vi "Create and Script 1553 System Definition.vi"(7 "configure logging":bool, 8 "error in":errorcluster, 11 "System Definition Name":string) -> (0 "error out":errorcluster, 2 "log file path":string, 3 "System Definition Path":path)   [LabVIEW 2023]
uses:
  Shared/AIM Hardware Parameters.ctl
  Shared/Initialization Method.ctl
  Shared/Bus Selection.ctl
  Shared/Coupling Mode.ctl
  Shared/Timing Mode.ctl
  <vilib>/NI/VeriStand Custom Device Testing Tools/VeriStandTestUtilities/VeriStandTestUtilities.lvlib
  Scripting/AIM MIL-STD-1553 Scripting.lvlib
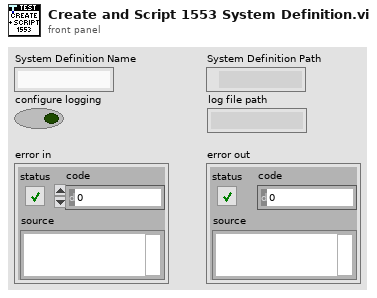
[diagram p1: front panel]
types:
  T1 = typedef "AIM Hardware Parameters.ctl" = cluster{"initialization method":T2, "card number":i32, "pxi slot number":i32, "biu number":i32, "bus selection":T3, "coupling mode":T4, "timing mode":T5}
  T2 = typedef "Initialization Method.ctl" = enum16{"PXI Slot Number", "Card Number"}
  T3 = typedef "Bus Selection.ctl" = enum16{"Both", "Primary", "Secondary"}
  T4 = typedef "Coupling Mode.ctl" = enum16{"Isolated Onboard Termination", "Transformer Coupled", "Direct Coupled", "External with Onboard Termination", "Onboard Digital Wrap-around"}
  T5 = typedef "Timing Mode.ctl" = enum16{"Disabled (Relative Timestamps)", "IRIG (Internal System Time)", "IRIG (External Timing Source)"}
  T6 = typedef "Custom Device API.lvlib/Custom Device Item Ref.ctl" = u64
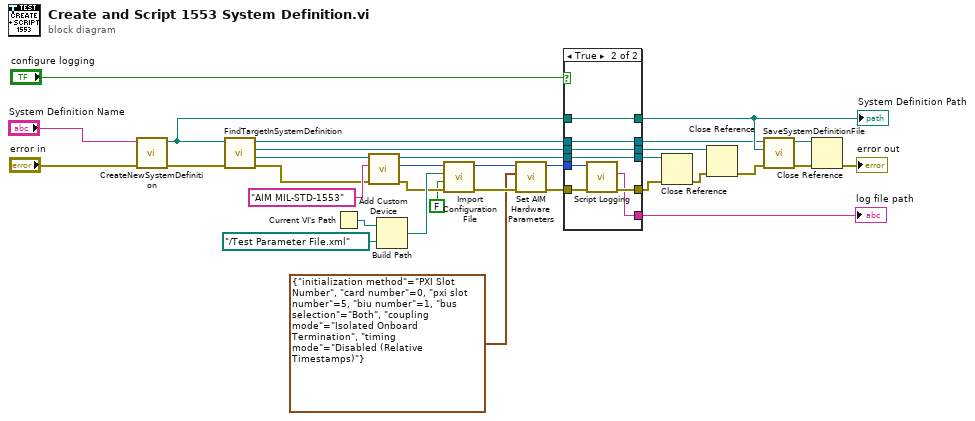
[diagram p0: block diagram]
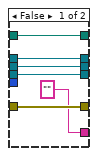
[diagram p2: hidden frame]
diagram:
  n1 = call <vilib>:"CreateNewSystemDefinition.vi"("error in"="error in", "System Definition Name"="System Definition Name") -> ("error out"=w16:errorcluster, "System Definition Path"=w8:path)  [unwired: 8 in]
  n2 = call <vilib>:"FindTargetInSystemDefinition.vi"("error in"=w16, "system definition path"=w8) -> ("error out"=w20:errorcluster, "Target"=w24:refnum<k24>, "Root"=w4:refnum<k24>, "System Definition"=w6:refnum<k24>)  [unwired: 6 in]
  n3 = Current VI's Path() -> (path=w15:path)
  n4 = call "Add Custom Device.vi"("error in"=w20, "custom device name"="AIM MIL-STD-1553" ("name"), "target"=w24) -> ("error out"=w26:errorcluster, "custom device"=w27:T6, "target out"=w3:refnum<k24>)  [unwired: 6 in]
  n5 = Build Path(base path=w15, name or relative path=path "../Test Parameter File.xml") -> (appended path=w29:path)
  n6 = call "Import Configuration File.vi"("error in"=w26, "create Tx/Rx folders for subaddresses?"=FALSE, "parameters configuration file path"=w29, "custom device"=w27) -> ("error out"=w31:errorcluster, "custom device out"=w32:T6)  [unwired: 6 in]
  n7 = call "Set AIM Hardware Parameters.vi"("error in"=w31, "aim hardware parameters"=T1 {"initialization method"=enum."PXI Slot Number", "card number"=0, "pxi slot number"=5, "biu number"=1, "bus selection"=enum."Both", "coupling mode"=enum."Isolated Onboard Termination", "timing mode"=enum."Disabled (Relative Timestamps)"} ("device parameters"), "custom device"=w32) -> ("error out"=w13:errorcluster, "custom device out"=w14:T6)  [unwired: 7 in]
  n8 = case shown="True" "configure logging" {
    tunnel: w14 -> [_ w47]
    tunnel: w13 -> [w39 w46]
    tunnel: [w39 w45] -> w12
    tunnel: ["" ("RT log file path") w44] -> w11
    tunnel: [w38 w43] -> w9
    tunnel: w8 -> [w38 w43]
    tunnel: [w37 w41] -> w7
    tunnel: w6 -> [w37 w41]
    tunnel: [w36 w42] -> w5
    tunnel: w4 -> [w36 w42]
    tunnel: w3 -> [w35 w40]
    tunnel: [w35 w40] -> w2
    frame False {
    }
    frame True {
      n9 = call "Script Logging.vi"("error in (no error)"=w46, "custom device"=w47) -> ("error out"=w45:errorcluster, "RT log file path"=w44:string)  [unwired: 7 in, 1 out]
    }
  }
  "System Definition Path" <- w9
  "log file path" <- w11
  n10 = Close Reference(reference=w2, error in (no error)=w12) -> (error out=w22:errorcluster)
  n11 = Close Reference(reference=w5, error in (no error)=w22) -> (error out=w23:errorcluster)
  n12 = call <vilib>:"SaveSystemDefinitionFile.vi"("error in (no error)"=w23, "System Definition File in"=w9, "System Definition Reference in"=w7) -> ("error out"=w19:errorcluster, "System Definition Reference out"=w18:refnum<k24>)  [unwired: 7 in]
  n13 = Close Reference(reference=w18, error in (no error)=w19) -> (error out=→"error out":errorcluster)
